vi "Set Acceleration.vi"(8 "error in (no error)":errorcluster, 9 "Acceleration":dbl, 10 "Axis Name":string, 11 "SIM Motion Controller in":refnum<class "Fine SIM Motion Controller.lvclass">) -> (0 "error out":errorcluster, 3 "SIM Motion Controller out":refnum<class "Fine SIM Motion Controller.lvclass">)   [LabVIEW 2022 SP3, in "Fine SIM Motion Controller.lvclass"]
uses:
  Fine SIM Motion Controller.lvclass
  Fine SIM Motion Controller.lvclass/Fine SIM Motion Controller.ctl
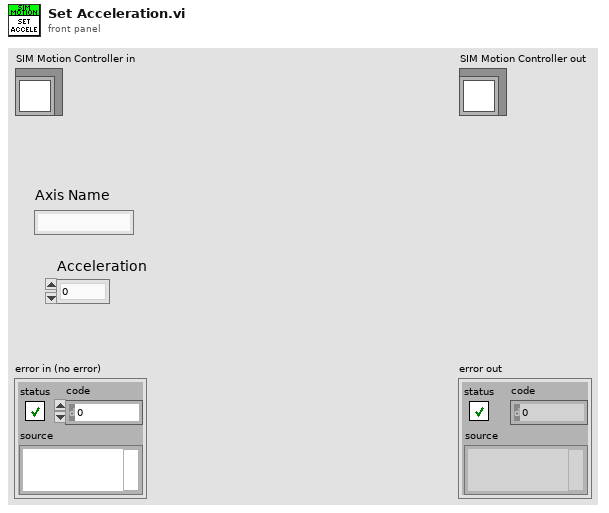
[diagram p1: front panel]
types:
  T1 = typedef "Parent SIM Motion Controller.lvclass/Axis Data.ctl" = cluster{"Axis Parameters":T2, "Axis Settings":T3, "Time Stamp":timestamp}
  T2 = typedef "Parent SIM Motion Controller.lvclass/Axis Parameters.ctl" = cluster{"Moving":bool, "Homed":bool, "Desired Position":dbl, "Current Positon":dbl, "Current Speed":dbl}
  T3 = typedef "Parent SIM Motion Controller.lvclass/Axis Settings.ctl" = cluster{"Speed":dbl, "Acceleration":dbl}
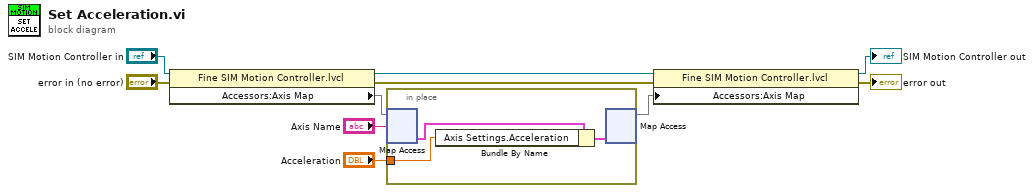
[diagram p0: block diagram]
diagram:
  n1 = property class="Fine SIM Motion Controller.lvcl"(reference="SIM Motion Controller in", error in="error in (no error)") -> (reference out=w9:refnum<class "Fine SIM Motion Controller.lvclass">, error out=w1:errorcluster, "Accessors:Axis Map"=w8:map{string, T1})
  n2 = in-place {
    in-place-border: "Acceleration" -> [w11]
    n3 = in-place-map #1(w8, "Axis Name") -> (w13:T1)  [unwired: 1 in, 1 out]
    n4 = Bundle By Name(cluster=w13, "Axis Settings.Acceleration"=w11) -> (w12:T1)
    n5 = in-place-map #1(w12) -> (w4:map{string, T1})  [unwired: 1 in, 2 out]
  }
  n6 = property class="Fine SIM Motion Controller.lvcl"(reference=w9, error in=w1, "Accessors:Axis Map"=w4) -> (reference out=→"SIM Motion Controller out":refnum<class "Fine SIM Motion Controller.lvclass">, error out=→"error out":errorcluster)
